vi "Update DatabaseF.vi"(0 "Frequency":string="40000057.37", 1 "connection information":path, 2 "Temperature":string, 3 "DC_SN":string) -> ()   [LabVIEW 2024]
uses:
  <vilib>/addons/database/Connection.llb/DB Tools Open Connec (Path).vi
  <vilib>/addons/database/Connection.llb/Conn Execute.vi
  <vilib>/addons/database/Recordset.llb/Rec Destroy - Connection.vi
  <vilib>/addons/database/_DB Variant To Data/Database Variant To Data.xnode
  <vilib>/addons/database/NI_Database_API.lvlib
panel:
  out "Time Measured":string
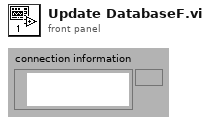
[diagram p1: front panel]
types:
  T1 = typedef "NI_Database_API.lvlib/Conn ObjectReference.ctl" = refnum<k1>
  T2 = typedef "NI_Database_API.lvlib/Rec ObjectReference.ctl" = refnum<k1>
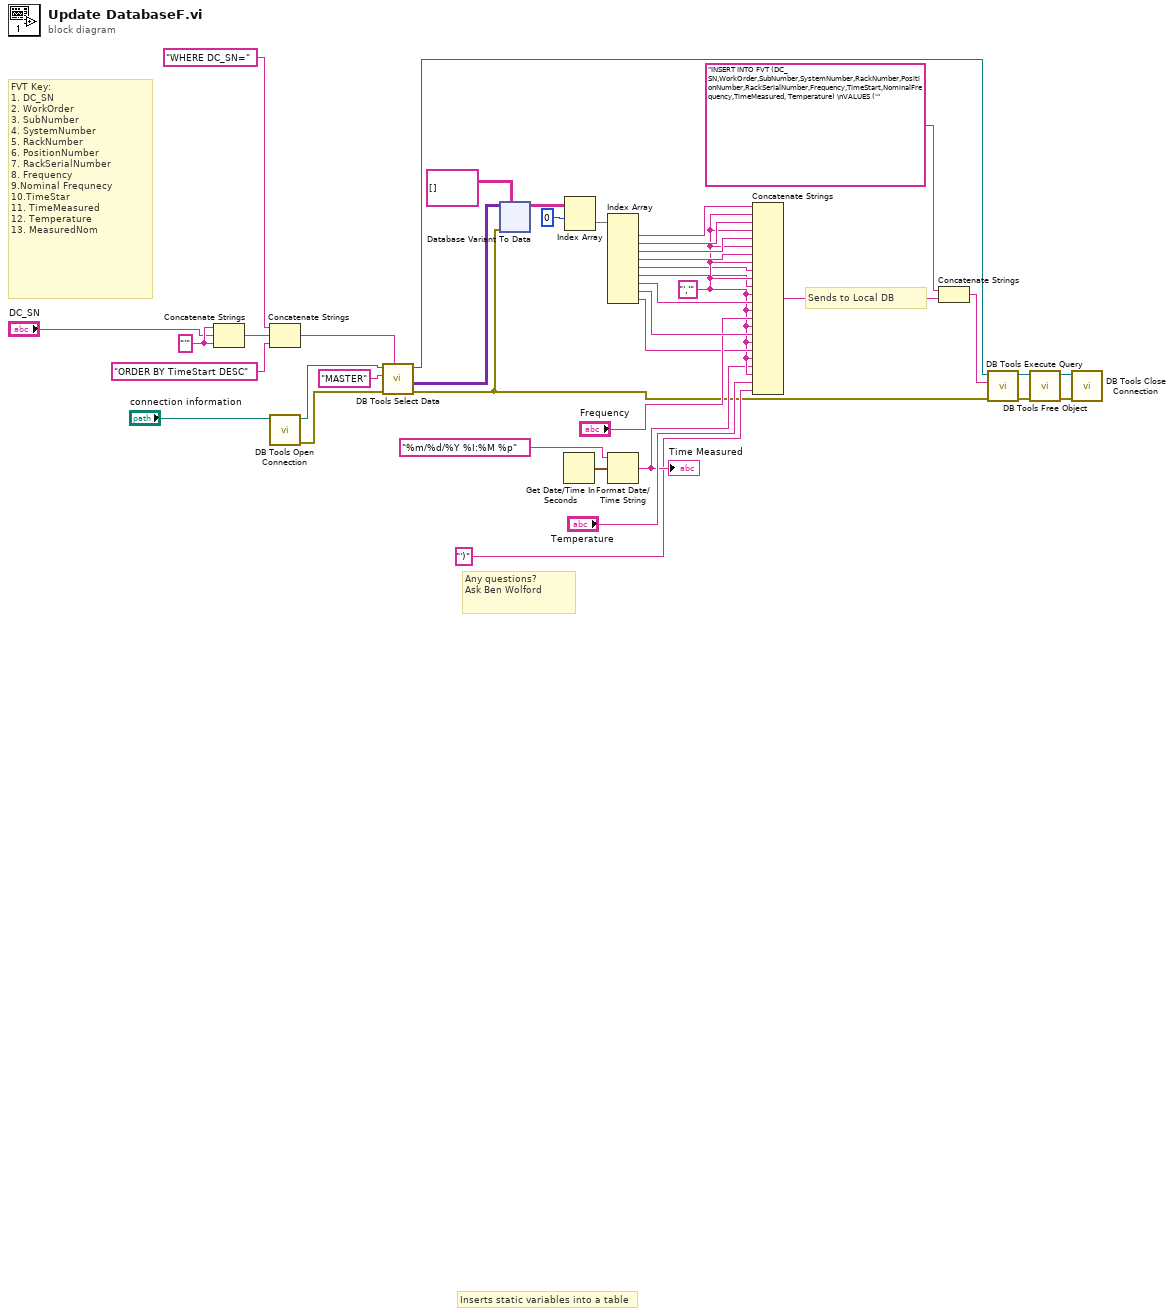
[diagram p0: block diagram]
diagram:
  w19 = "'" ("string")
  w27 = "','"
  # "Sends to Local DB"
  # "Inserts static variables into a table"
  # "FVT Key:\n1. DC_SN\n2. WorkOrder\n3. SubNumber\n4. SystemNumber\n5. RackNumber\n6. PositionNumber\n7. RackSerialNumber\n8. Frequency\n9.Nominal Frequnecy\n10.TimeStar\n11. TimeMeasured\n12. Temperature\n13. MeasuredNom"
  # "Any questions? \nAsk Ben Wolford"
  n1 = Concatenate Strings(w19, "DC_SN", w19) -> (w18:string)
  n2 = Concatenate Strings("WHERE DC_SN=" ("SQL Query"), w18, "ORDER BY TimeStart DESC" ("string")) -> (w11:string)
  n3 = call-poly <vilib>:"DB Tools Open Connection.vi"("connection information"="connection information") -> ("error out"=w15:errorcluster, "connection reference"=w14:T1)  [unwired: 7 in]
  n4 = call <vilib>:"DB Tools Select Data.vi"("condition"=w11, "error in (no error)"=w15, "table"="MASTER", "connection reference"=w14) -> ("error out"=w2:errorcluster, "data"=w16:variant[][], "connection reference out"=w3:T1)  [unwired: 2 in]
  n5 = xnode "Database Variant To Data"("database variant"=w16, "error in (no error)"=w2, "type"=string[][] []) -> ("data"=w10:string[][])  [unwired: 1 out]
  n6 = Get Date/Time In Seconds() -> (seconds since 1Jan1904=w38:timestamp)
  n7 = Index Array(array=w10, index (row)=0 ("disabled index (row)")) -> (element=w9:string[])  [unwired: 1 in]
  n8 = Index Array(array=w9) -> (element #1=w36:string, element #2=w35:string, element #3=w34:string, element #4=w33:string, element #5=w26:string, element #6=w25:string, element #7=w32:string, element #8=w40:string, element #9=w28:string)  [unwired: 9 in]
  n9 = Format Date/Time String(time format string (%c)="%m/%d/%Y %I:%M %p", seconds (now)=w38) -> (date/time string=w24:string)  [unwired: 1 in]
  "Time Measured" <- w24
  n10 = Concatenate Strings(w36, w27, w35, w27, w34, w27, w33, w27, w26, w27, w25, w27, w32, w27, "Frequency", w27, w40, w27, w28, w27, w24, w27, "Temperature", "')" ("string")) -> (w39:string)
  n11 = Concatenate Strings("INSERT INTO FVT (DC_SN,WorkOrder,SubNumber,SystemNumber,RackNumber,PositionNumber,RackSerialNumber,Frequency,TimeStart,NominalFrequency,TimeMeasured, Temperature) \nVALUES ('" ("string"), w39) -> (w1:string)
  n12 = call-poly <vilib>:"DB Tools Execute Query.vi"("error in (no error)"=w2, "SQL query"=w1, "connection reference"=w3) -> ("error out"=w5:errorcluster, "recordset reference"=w4:T2)  [unwired: 5 in]
  n13 = call-poly <vilib>:"DB Tools Free Object.vi"("error in (no error)"=w5, "recordset reference"=w4) -> ("error out"=w7:errorcluster, "connection reference"=w6:T1)  [unwired: 8 in]
  n14 = call <vilib>:"DB Tools Close Connection.vi"("error in (no error)"=w7, "connection reference"=w6) -> ()  [unwired: 5 in, 1 out]
